vi "Y5140_SetCurr.vi"(8 "error in (no error)":errorcluster caption="错误输入（无错误）", 11 "MyIndex":u8) -> (0 "error out":errorcluster caption="错误输出", 1 "T/F":bool, 2 "Value":sgl)   [LabVIEW 2015]
uses:
  <vilib>/Instr/_visa.llb/VISA Configure Serial Port (Instr).vi
panel:
  out "VISA":refnum<visa-resource-name> caption="VISA资源名称输出"
  in  "设置电流值(A)":dbl=1.0
  out "Rx":string
  out "Tx":string
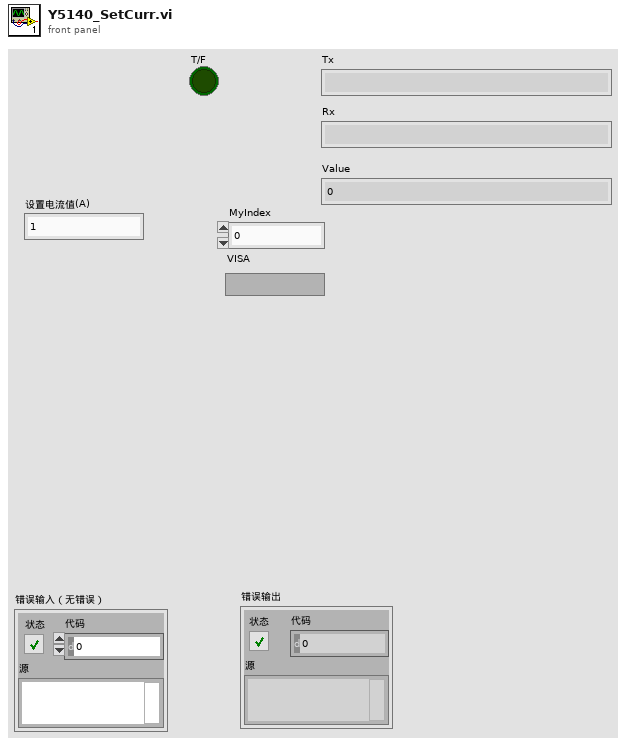
[diagram p1: front panel]
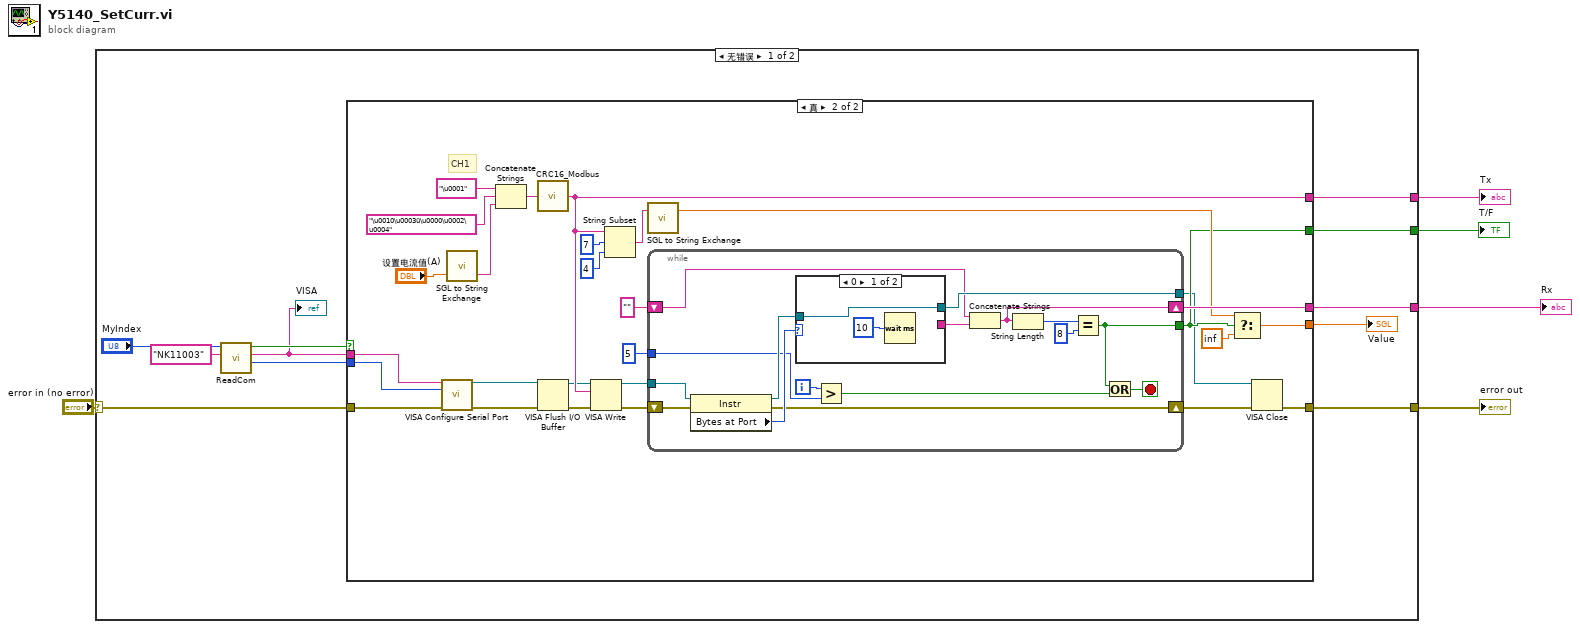
[diagram p0: block diagram]
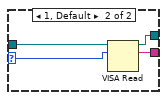
[diagram p3: hidden frame]
diagram:
  n1 = case shown="无错误" "error in (no error)" {
    selector: "error in (no error)" -> [w15 w67]
    tunnel: [w14 w67] -> w4
    tunnel: [w13 _] -> w3
    tunnel: [w12 _] -> w2
    tunnel: [w11 _] -> w1
    frame No Error {
      n2 = call "ReadCom.vi"("仪器名称"="NK11003", "MyIndex"="MyIndex") -> ("Baudrate"=w6:i32, "COM"=w7:string, "OK?"=w8:bool)  [unwired: 7 in]
      "VISA" <- w7
      n3 = case shown="真" w8 {
        tunnel: [_ w44] -> w16
        tunnel: w15 -> [_ w43]
        tunnel: [_ w18] -> w14
        tunnel: [_ w41] -> w13
        tunnel: [_ w39] -> w12
        tunnel: [_ w23] -> w11
        tunnel: w7 -> [_ w21]
        tunnel: w6 -> [_ w20]
        frame False {
        }
        frame True {
          # "CH1"
          n4 = call-poly "VISA Configure Serial Port"("VISA resource name"=w21, "baud rate (9600)"=w20, "error in (no error)"=w43) -> ("VISA resource name out"=w19:refnum<visa-resource-name>, "error out"=w22:errorcluster)  [unwired: 11 in]
          n5 = call "SGL to String Exchange.vi"("SGL In"="设置电流值(A)") -> ("4字节字符串"=w24:string)  [unwired: 1 in, 1 out]
          n6 = Concatenate Strings("\u0001", "\u0010\u0003ü\u0000\u0002\u0004", w24) -> (w25:string)
          n7 = call "CRC16_Modbus.vi"("需要校验的数据"=w25) -> ("String+CRC16"=w41:string)
          n8 = VISA Flush I/O Buffer(VISA resource name=w19, error in (no error)=w22) -> (VISA resource name out=w37:refnum<visa-resource-name>, error out=w36:errorcluster)  [unwired: 1 in]
          n9 = VISA Write(VISA resource name=w37, write buffer=w41, error in (no error)=w36) -> (VISA resource name out=w35:refnum<visa-resource-name>, error out=w34:errorcluster)  [unwired: 1 out]
          n10 = String Subset(string=w41, offset (0)=7 ("偏移量(0)"), length (rest)=4 ("长度（剩余）")) -> (substring=w29:string)
          n11 = call "SGL to String Exchange.vi"("4字节字符串"=w29) -> ("IEE754Floatout"=w28:sgl)  [unwired: 1 in, 1 out]
          n12 = while {
            tunnel: w35 -> [w60]
            tunnel: [w57] -> w17
            shift-right: [w49] -> w39
            shift-left: "" -> [w55]
            tunnel: 5 ("y") -> [w53]
            tunnel: [w45] -> w23
            shift-right: [w51] -> w42
            shift-left: w34 -> [w52]
            i -> [w54]
            stop <- w46 stop-if-true
            n13 = property class="Instr"(reference=w60, error in=w52) -> (reference out=w58:refnum<visa-resource-name>, error out=w51:errorcluster, "Bytes at Port"=w59:u32)
            n14 = case shown="0" w59 {
              selector: w59 -> [_ w65]
              tunnel: w58 -> [w62 w66]
              tunnel: [w62 w64] -> w57
              tunnel: [_ w63] -> w56
              frame 0 {
                n15 = Wait (ms)(milliseconds to wait=u32 10 ("等待时间（毫秒）")) -> ()  [unwired: 1 out]
              }
              frame 1, Default {
                n16 = VISA Read(VISA resource name=w66, byte count=w65) -> (VISA resource name out=w64:refnum<visa-resource-name>, read buffer=w63:string)  [unwired: 1 in, 2 out]
              }
            }
            n17 = Greater?(x=w54, y=w53) -> (0:w50:bool)
            n18 = Concatenate Strings(w55, w56) -> (w49:string)
            n19 = String Length(string=w49) -> (length=w48:i32)
            n20 = Equal?(x=w48, y=8) -> (x = y?=w45:bool)
            n21 = Or(x=w45, y=w50) -> (x .or. y?=w46:bool)
          }
          n22 = Select(t=w28, s=w23, f=sgl inf) -> (s? t:f=w44:sgl)
          n23 = VISA Close(VISA resource name=w17, error in (no error)=w42) -> (error out=w18:errorcluster)
        }
      }
      "Value" <- w16
    }
    frame Error {
    }
  }
  "error out" <- w4
  "Tx" <- w3
  "Rx" <- w2
  "T/F" <- w1
